vi "CUSTOM_UI.vi"() -> ()   [LabVIEW 2023]
panel:
  in  "Boolean 2":bool
  in  "Boolean":bool
  out "Gauge":dbl(knob) scale=0.0..10.0
  in  "Vertical Pointer Slide":dbl(slide) scale=0.0..10.0
  in  "Tank":dbl(slide) scale=0.0..10.0
  in  "Listbox":i32(listbox)
  in  "Button":bool
  in  "Combo Box 2":string(combo)
  in  "String":string
  in  "Numeric":dbl
  in  "Path":path
  out "Waveform Graph":waveform(dbl)(graph)
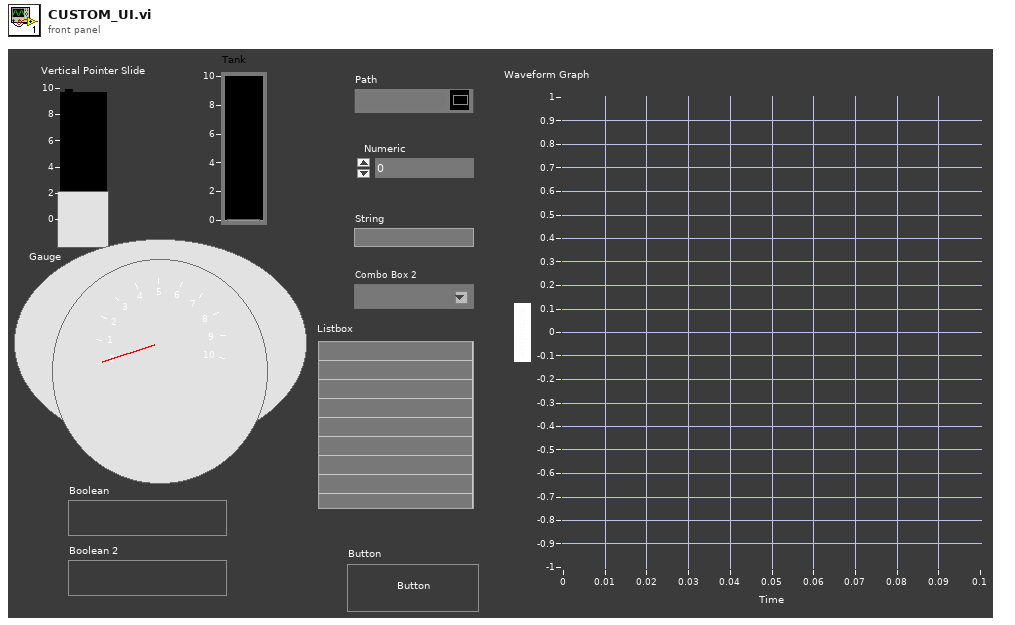
[diagram p1: front panel]
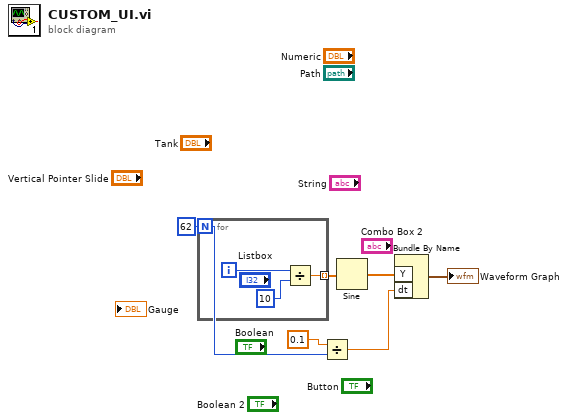
[diagram p0: block diagram]
diagram:
  w4 = 62
  n1 = for {
    N: w4 -> [_]
    tunnel: [w7] -> w6 mode=indexing
    i -> [w9]
    n2 = Divide(x=w9, y=10) -> (x/y=w7:dbl)
  }
  n3 = Divide(x=0.1 ("y"), y=w4) -> (x/y=w2:dbl)
  n4 = Sine(x=w6) -> (sin(x)=w5:dbl[])
  n5 = Bundle By Name("Y"=w5, "dt"=w2) -> (→"Waveform Graph":waveform(dbl))  [unwired: 1 in]
